vi "Write Startup Model-View Configuration.vi"(7 "Application Style":refnum<class "IApplicationStyle.lvclass">, 8 "Mediator Type":refnum<class "IMediator.lvclass">, 9 "Model Type":refnum<class "IModel.lvclass">, 10 "Startup View Configuration":refnum<class "IViewable.lvclass">, 11 "IViewModel In":refnum<class "IViewModel.lvclass">) -> (3 "IViewModel Out":refnum<class "IViewModel.lvclass">)   [LabVIEW 2017, in "IViewModel.lvlib" / "IViewModel.lvclass"]
doc: "This constructor is only deprecated for public calls. It should be replaced with the malleable \"Construct MVA Application.vim\" which extends by adding optional framework-level event logging to one or more sinks."
uses:
  IViewModel.lvclass
  C:/Git/mva-framework/Source/Framework/IViewManager/IViewManager/IViewManager.lvclass
  IViewable/IViewable/IViewable.lvclass
  IModel/IModel/IModel.lvclass
  IMediator/IMediator/IMediator.lvclass
  IViewable/IApplicationStyle/IApplicationStyle.lvclass
  IViewModel.lvclass/IViewModel.ctl
  IViewManager/IViewManager Messages/Launch Nested Views Msg/Launch Nested Views Msg.lvclass/Launch Nested Views Msg.ctl
  IViewManager/IViewManager/IViewManager.lvclass/IViewManager.ctl
  IViewManager/IViewManager Messages/Launch Nested Views Msg/Launch Nested Views Msg.lvclass
  IViewManager/IViewManager/IViewManager.lvclass
panel:
  # "Replace public calls of this method with\nConstruct MVA Application.vim"
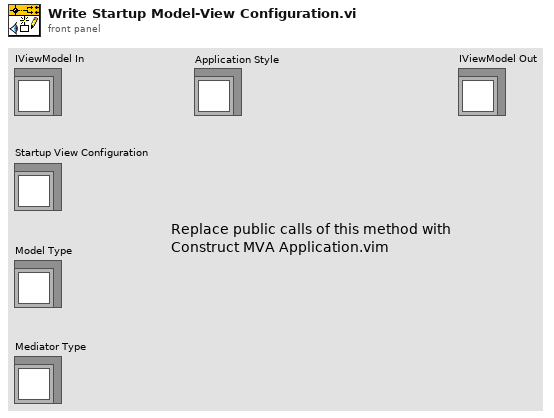
[diagram p1: front panel]
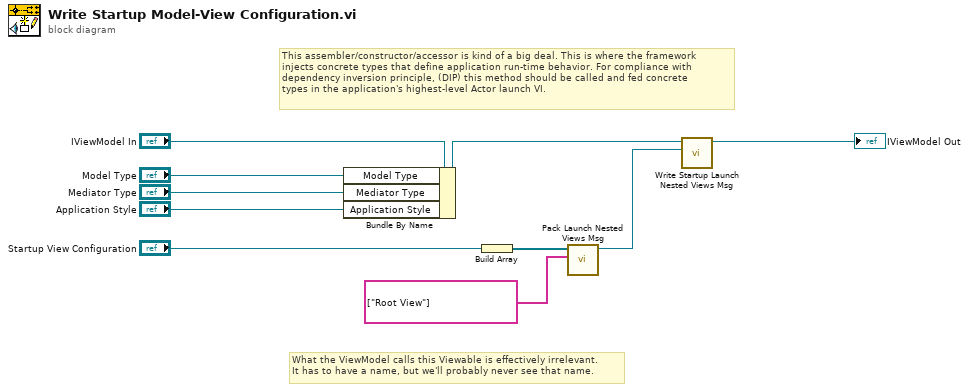
[diagram p0: block diagram]
diagram:
  # "This assembler/constructor/accessor is kind of a big deal. This is where the framework\ninjects concrete types that define application run-time behavior. For compliance with\ndependency inversion principle, (DIP) this method should be called and fed concrete\ntypes in the application's highest-level Actor launch VI."
  # "What the ViewModel calls this Viewable is effectively irrelevant.\nIt has to have a name, but we'll probably never see that name."
  n1 = Bundle By Name(cluster="IViewModel In", "Model Type"="Model Type", "Mediator Type"="Mediator Type", "Application Style"="Application Style") -> (w4:refnum<class "IViewModel.lvclass">)
  n2 = Build Array("Startup View Configuration") -> (w8:refnum<class "IViewable.lvclass">[])
  n3 = call "Pack Launch Nested Views Msg.vi"("View Labels"=string[] ["Root View"] ("View Labels (optional)"), "Nested Views"=w8) -> ("Launch Nested Views Msg"=w6:refnum<class "Launch Nested Views Msg.lvclass">)  [unwired: 9 in]
  n4 = call "Write Startup Launch Nested Views Msg.vi"("Launch Nested Views Msg"=w6, "IViewManager in"=w4) -> ("IViewManager out"=→"IViewModel Out":refnum<class "IViewModel.lvclass">)  [unwired: 9 in]
